vi "Configure GPIB Address.vi"(8 "error in (no error)":errorcluster, 10 "GPIB Address (26)":i32=26, 11 "VISA resource name":refnum<visa-resource-name>) -> (0 "error out":errorcluster, 3 "VISA resource name out":refnum<visa-resource-name>)   [LabVIEW 2015, in "Keithley 2600 Series.lvlib"]
doc: "Configures the GPIB address.\n\n<b>Note:</b>\n(1) This VI is not available on the models 2606B.\n(2) The GPIB address is stored in nonvolatile memory. The <b>SMU Reset</b> VI has no affect on the address."
uses:
  Keithley 2600 Series.lvlib
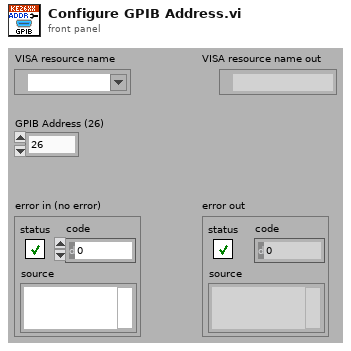
[diagram p1: front panel]
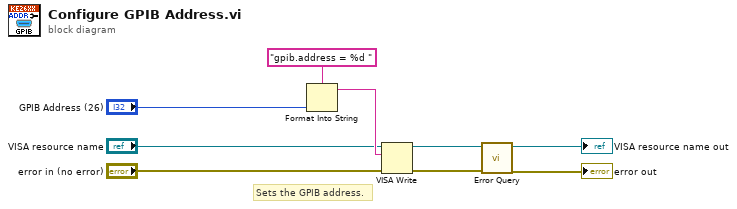
[diagram p0: block diagram]
diagram:
  # "Sets the GPIB address."
  n1 = Format Into String(format string="gpib.address = %d ", "GPIB Address (26)") -> (resulting string=w7:string)  [unwired: 2 in, 1 out]
  n2 = VISA Write(VISA resource name="VISA resource name", write buffer=w7, error in (no error)="error in (no error)") -> (VISA resource name out=w4:refnum<visa-resource-name>, error out=w3:errorcluster)  [unwired: 1 out]
  n3 = call "Error Query.vi"("error in (no error)"=w3, "VISA resource name"=w4) -> ("error out"=→"error out":errorcluster, "VISA resource name out"=→"VISA resource name out":refnum<visa-resource-name>)  [unwired: 6 in, 2 out]
